vi "SQLite Query - Update.vi"(6 "A[Strings] Value":string[](array[string]), 7 "A[Strings]":string[](array[string]), 8 "error in":errorcluster, 9 "Data":string[](array[string]), 10 "Table Headers":string[](array[string]), 11 "Table Name":string) -> (0 "error out":errorcluster, 3 "SQLite Query":string="UPDATE 'LVData' SET 'Numeric Data'=57,'Float Data'=12.540000,'String Data'='TesSolve','Enum Data'='Enum Item 1','Array Data[0].Numeric Data'=1,'Array Data[1].Numeric Data'=4,'Array Data[2].Numeric Data'=7,'Array Data[3].Numeric Data'=8,'Array Data[4].Numeric Data'=1,'Array Data 2[0].Numeric Data'=1,'Array Data 2[1].Numeric Data'=2 WHERE \"Numeric Data\"='401' AND\"String Data\"='q';")   [LabVIEW 2014, in "TableLogger_SQLite_Actor.lvlib" / "TableLogger_SQLite_Actor.lvclass"]
uses:
  TableLogger_SQLite_Actor.lvclass
  <userlib>/_OpenG.lib/array/array.llb/Remove Duplicates from 1D Array (String)__ogtk.vi
  TableLogger_CSV_Actor/TableLogger_CSV_Actor/TableLogger_CSV_Actor.lvclass
panel:
  # "Connector Pane"
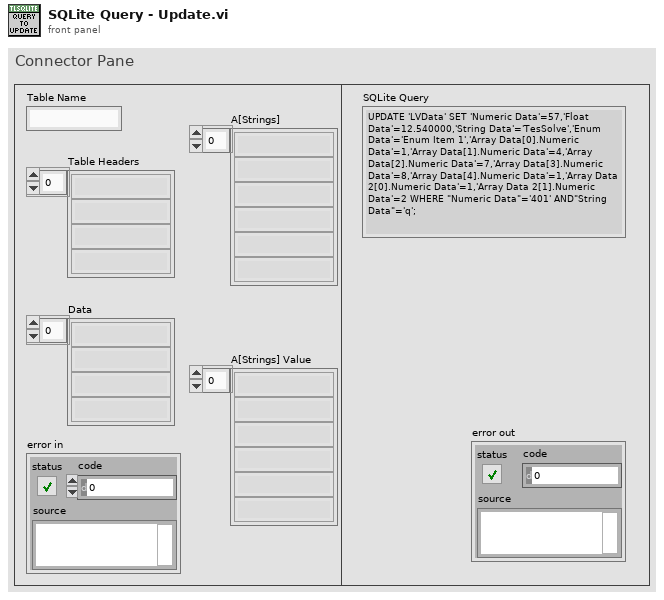
[diagram p1: front panel]
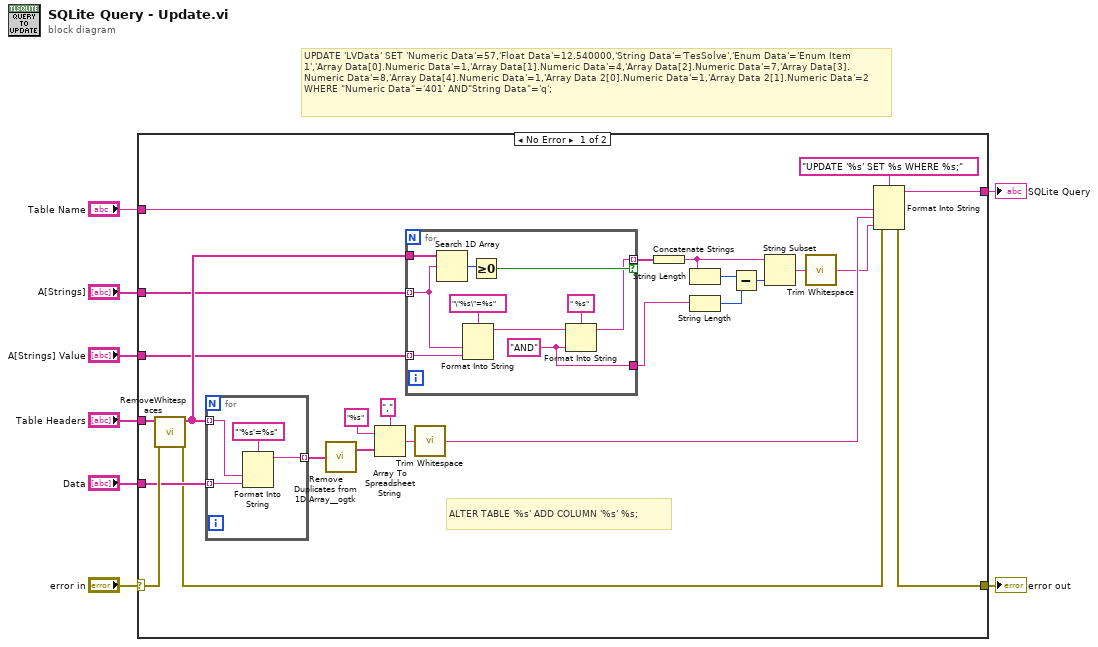
[diagram p0: block diagram]
diagram:
  # "UPDATE 'LVData' SET 'Numeric Data'=57,'Float Data'=12.540000,'String Data'='TesSolve','Enum Data'='Enum Item 1','Array Data[0].Numeric Data'=1,'Array Data[1].Numeric Data'=4,'Array Data[2].Numeric Data'=7,'Array Data[3].Numeric Data'=8,'Array Data[4].Numeric Data'=1,'Array Data 2[0].Numeric Data'=1,'Array Data 2[1].Numeric Data'=2 WHERE \"Numeric Data\"='401' AND\"String Data\"='q';"
  n1 = case shown="No Error" "error in" {
    selector: "error in" -> [w32 w48]
    tunnel: "Data" -> [w24 _]
    tunnel: "Table Name" -> [w23 _]
    tunnel: "Table Headers" -> [w33 _]
    tunnel: [w10 w48] -> w4
    tunnel: [w22 _] -> w3
    tunnel: "A[Strings]" -> [w13 _]
    tunnel: "A[Strings] Value" -> [w12 _]
    frame No Error {
      # "ALTER TABLE '%s' ADD COLUMN '%s' %s;"
      n2 = call "RemoveWhitespaces.vi"("error in (no error)"=w32, "Array In"=w33) -> ("error out"=w11:errorcluster, "Array removing empty space"=w14:string[])  [unwired: 8 in]
      n3 = for {
        tunnel: w14 -> [w46] mode=indexing
        tunnel: w24 -> [w44] mode=indexing
        tunnel: [w45] -> w29 mode=indexing
        n4 = Format Into String(format string="'%s'=%s", w46, w44) -> (resulting string=w45:string)  [unwired: 2 in, 1 out]
      }
      n5 = call-poly <userlib>:"Remove Duplicates from 1D Array__ogtk.vi"("Input Array"=w29) -> ("Output Array"=w27:string[])  [unwired: 1 out]
      n6 = Array To Spreadsheet String(delimiter (Tab)=",", array=w27, 3:"%s" ("format string")) -> (spreadsheet string=w30:string)
      n7 = for {
        tunnel: w14 -> [w43]
        tunnel: w13 -> [w38] mode=indexing
        tunnel: w12 -> [w39] mode=indexing
        tunnel: [w36] -> w17 mode=indexing if=w41
        tunnel: [w34] -> w16
        w34 = "AND" ("input 1")
        n8 = Search 1D Array(1D array=w43, element=w38) -> (index of element=w42:i32)  [unwired: 1 in]
        n9 = Format Into String(format string="\"%s\"=%s", w38, w39) -> (resulting string=w37:string)  [unwired: 2 in, 1 out]
        n10 = Greater Or Equal To 0?(x=w42) -> (x >= 0?=w41:bool)
        n11 = Format Into String(format string=" %s", initial string=w37, w34) -> (resulting string=w36:string)  [unwired: 1 in, 1 out]
      }
      n12 = call <vilib>:"Trim Whitespace.vi"("string"=w30) -> ("trimmed string"=w31:string)  [unwired: 1 in]
      n13 = Concatenate Strings(w17) -> (w19:string)
      n14 = String Length(string=w19) -> (length=w20:i32)
      n15 = String Length(string=w16) -> (length=w15:i32)
      n16 = Subtract(x=w20, y=w15) -> (x-y=w21:i32)
      n17 = String Subset(string=w19, length (rest)=w21) -> (substring=w18:string)  [unwired: 1 in]
      n18 = call <vilib>:"Trim Whitespace.vi"("string"=w18) -> ("trimmed string"=w9:string)  [unwired: 1 in]
      n19 = Format Into String(format string="UPDATE '%s' SET %s WHERE %s;" ("SQL"), error in=w11, w23, w31, w9) -> (resulting string=w22:string, error out=w10:errorcluster)  [unwired: 1 in]
    }
    frame Error {
    }
  }
  "SQLite Query" <- w3
  "error out" <- w4
